vi "Drivebase Controller.vi"(8 "error in":errorcluster) -> ()   [LabVIEW 2019]
doc: "This VI executes continuously carrying out the current operation and responding to updates or new operations. It will often contain the timing or control code that is difficult to place directly in TeleOp. This VI generally opens all sensors and motors and isolates the rest of the robot code from knowing how the operations are carried out."
uses:
  <vilib>/Rock Robotics/WPI/Framework/Completion Status.ctl
  Drivebase Setpoints.ctl
  Drivebase Operations.ctl
  Bordeaux/bordeaux-pathinator/Bordeaux/Command Stuff/Single Cmd Info.ctl
  <vilib>/picture/picture.llb/imagedata.ctl
  <vilib>/Rock Robotics/WPI/ThirdParty/REV Robotics/SPARK MAX/Typedef/Spark MAX Idle Mode.ctl
  IMU/Typedef/ADIS16470 Data.ctl
  <vilib>/Rock Robotics/WPI/ThirdParty/REV Robotics/SPARK MAX/Typedef/Spark MAX Control Type.ctl
  Framework/Robot Global Data.vi
panel:
  out "x-y":u32(graph)
  out "timing delay err 2":dbl(graph)
  in  "Interactive Values":T1
  out "Current\nCmd":string
  in  "Buttons":cluster{"Execute Cmd":bool, "Abort Cmd":bool}
  out "Command Timing":cluster{"Start Time (ms)":u32, "Iterations":i32}
  out "Status":T5
  # "Tip: It may be helpful to observe inputs and sensor values.\nYou may also want to display tuning or debugging controls."
  # "Interactive Command: You may fill in the settings for a command\nand schedule it with the Execute button. You can observe and abort\nany command while fine tuning the code for the controller."
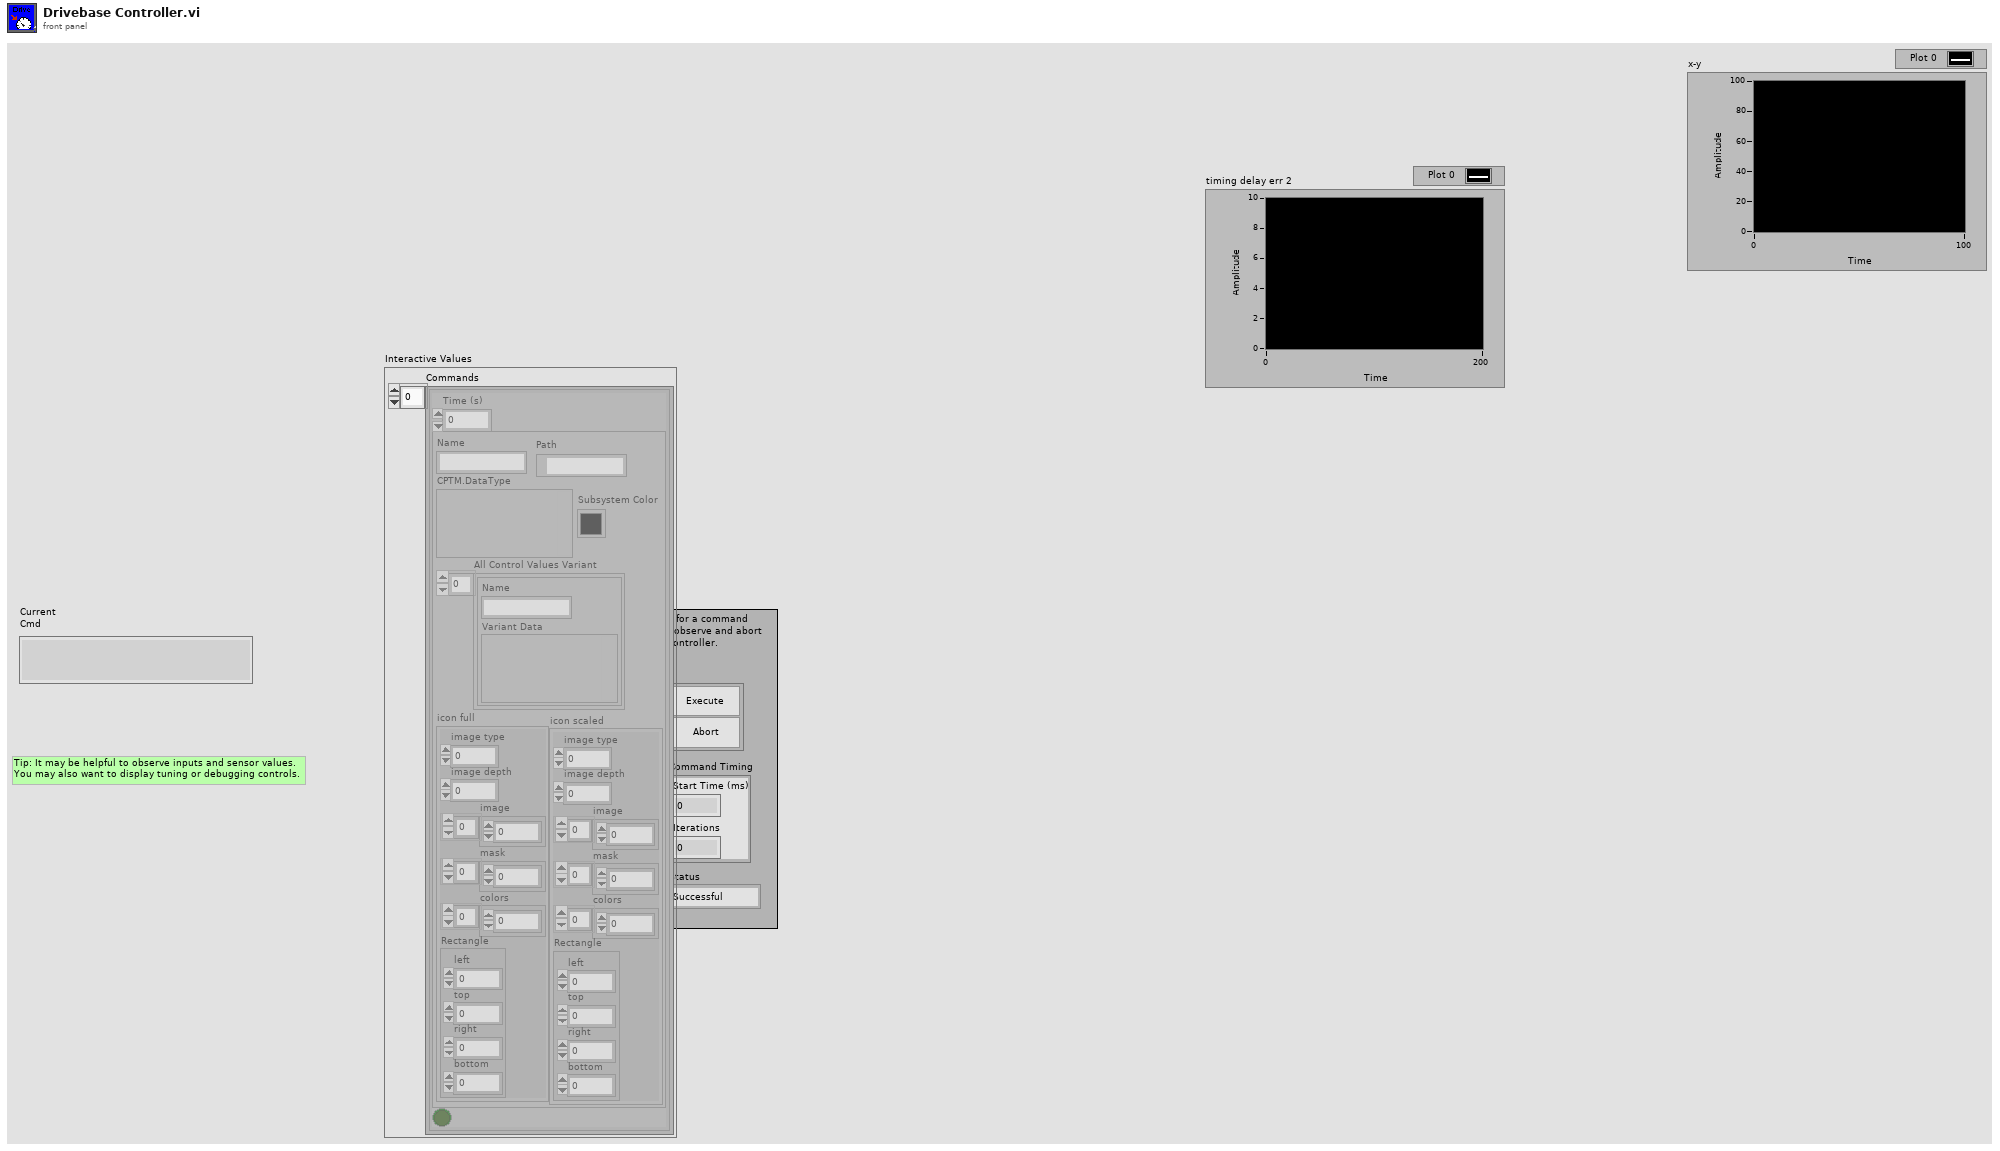
[diagram p1: front panel]
types:
  T1 = typedef "Drivebase Setpoints.ctl" = cluster{"Operation":T2, "Left Setpoint":dbl, "Right Setpoint":dbl, "Velocity":dbl[], "Angles":dbl[], "Reset Gyro":bool, "Booleans":cluster{"Robot Backwards":bool, "Path Backwards":bool}, "Commands":cluster{"Time (s)":dbl, T3, bool}[]}
  T2 = typedef "Drivebase Operations.ctl" = enum16{"Reserve", "Read Current", "Immediate", "Pathinator"}
  T3 = typedef "Single Cmd Info.ctl" = cluster{"Name":string, "CPTM.DataType":variant, "All Control Values Variant":cluster{"Name":string, "Variant Data":variant}[], "icon full":T4, "icon scaled":T4, "Path":path, "Subsystem Color":u32}
  T4 = typedef "imagedata.ctl" = cluster{"image type":i32, "image depth":i32, "image":u8[], "mask":u8[], "colors":u32[], "Rectangle":cluster{"left":i16, "top":i16, "right":i16, "bottom":i16}}
  T5 = typedef "Completion Status.ctl" = enum16{"Successful", "Aborted", "Incomplete"}
  T6 = cluster{"P Gain":dbl, "I Gain":dbl, "D Gain":dbl, "F Gain":dbl, "I Zone":dbl, "Min Output":dbl, "Max Output":dbl}
  T7 = typedef "Spark MAX Idle Mode.ctl" = enum16{"Coast", "Brake"}
  T8 = typedef "WPI_MotorControlDeviceRef.ctl" = cluster{"DeviceStatus":errorcluster, "Type":T9, "PWM":cluster{"PWM Channel":T10, "DeadBand":T11}, "CAN":cluster{"Device Number":u8, "SetOutput VI Ref":variant, "GetOutput VI Ref":variant, "Enable VI Ref":variant, "Disable VI Ref":variant, "Data":variant}, "Invert":bool, "DIO PWM":cluster{"PWM \"Enable\" Channel":T10, "DIOChannel":T12, "PWM Rate":dbl}}
  T9 = typedef "WPI_MotorControlType.ctl" = enum16{"PWM", "CAN", "DIO PWM"}
  T10 = typedef "FPGA_DIOPWMChannel.ctl" = enum8{"PWM 0", "PWM 1", "PWM 2", "PWM 3", "PWM 4", "PWM 5", "PWM 6", "PWM 7", "PWM 8", "PWM 9", "PWM MXP 0", "PWM MXP 1", "PWM MXP 2", "PWM MXP 3", "PWM MXP 4", "PWM MXP 5", "PWM MXP 6", "PWM MXP 7", "PWM MXP 8", "PWM MXP 9", "Invalid"}
  T11 = typedef "WPI_PWMDeadband.ctl" = cluster{"Name":string, "maxPositivePwm":i32, "minPositivePwm":i32, "centerPwm":i32, "maxNegativePwm":i32, "minNegativePwm":i32, "angularRange":u16}
  T12 = typedef "FPGA_DIOChannel.ctl" = enum8{"DIO 0", "DIO 1", "DIO 2", "DIO 3", "DIO 4", "DIO 5", "DIO 6", "DIO 7", "DIO 8", "DIO 9", "DIO MXP 0", "DIO MXP 1", "DIO MXP 2", "DIO MXP 3", "DIO MXP 4", "DIO MXP 5", "DIO MXP 6", "DIO MXP 7", "DIO MXP 8", "DIO MXP 9", "DIO MXP 10", "DIO MXP 11", "DIO MXP 12", "DIO MXP 13", "DIO MXP 14", "DIO MXP 15", "SPI Port CS1", "SPI Port CS2", "SPI Port CS3", "SPI Port MISO", "SPI Port MOSI", "Invalid"}
  T13 = typedef "ADIS16470 Device Reference.ctl" = cluster{"DevStatus":errorcluster, "Hardware Config":T14, "Calibration Complete":refnum<notifier>, "Status FIFO":refnum<k33>, "Last Value Reference":refnum<data-value>, "Sychronous Process VI":T17, "Cmd FIFO":refnum<k33>, "Source":T18, "Data FIFO":refnum<k33>, "Calibration Time":T22}
  T14 = typedef "ADIS16470 Hardware Configuration.ctl" = cluster{"SPI Clock Rate (Hz)":dbl, "IMU SPI Mode (3)":T15, "IMU Reset Pin":T12, "IMU SPI Bus":T16, "IMU Data Ready Pin":T12, "Stall Config":cluster{"Pow2BytesPerRead":u8, "StallTicks":u16, "CsToSclkTicks":u8}}
  T15 = typedef "WPI_SPIMode.ctl" = enum16{"Mode 0 (Clk Idle Low,Sample on Leading)", "Mode 1 (Clk Idle Low,Sample on Trailing)", "Mode 2 (Clk Idle High,Sample on Leading)", "Mode 3 (Clk Idle High,Sample on Trailing)"}
  T16 = typedef "spi_bus.ctl" = enum16{"SPI On-Board, CS0", "SPI On-Board, CS1", "SPI On-Board, CS2", "SPI On-Board, CS3", "SPI MXP", "Invalid"}
  T17 = typedef "ADIS16470 Process.ctl" = refnum<vi>
  T18 = typedef "FPGA_CounterEncoderSourceConvertionLVSourceType.ctl" = cluster{"DevStatus":errorcluster, "AnalogTriggerMode?":bool, "DigitalMode":cluster{"DIO Channel":T19}, "AnalogTriggerMode":cluster{"AnalogTriggerIndex":T20, "OutputType":T21}}
  T19 = typedef "FPGA_DIODigitalSourceChannel.ctl" = enum8{"DIO 0", "DIO 1", "DIO 2", "DIO 3", "DIO 4", "DIO 5", "DIO 6", "DIO 7", "DIO 8", "DIO 9", "DIO MXP 0", "DIO MXP 1", "DIO MXP 2", "DIO MXP 3", "DIO MXP 4", "DIO MXP 5", "DIO MXP 6", "DIO MXP 7", "DIO MXP 8", "DIO MXP 9", "DIO MXP 10", "DIO MXP 11", "DIO MXP 12", "DIO MXP 13", "DIO MXP 14", "DIO MXP 15", "SPI Port CS1", "SPI Port CS2", "SPI Port CS3", "SPI Port MISO", "SPI Port MOSI", "Disabled"}
  T20 = typedef "FPGA_AnalogTriggerIndex.ctl" = enum8{"Trig 0", "Trig 1", "Trig 2", "Trig 3", "Trig 4", "Trig 5", "Trig 6", "Trig 7", "Invalid"}
  T21 = typedef "FPGA_AnalogTriggerOutType.ctl" = enum16{"InWindow", "TriggerState", "Rising", "Falling"}
  T22 = typedef "ADIS16470 Calibration Time.ctl" = enum16{"32ms", "64ms", "128ms", "256ms", "512ms", "1s", "2s", "4s", "8s", "16s", "32s", "64s"}
  T23 = typedef "Command Status Info.ctl" = cluster{"Name":string, "Status":T5, "notifier out":T24}
  T24 = typedef "Completion Notifier.ctl" = refnum<notifier>
  T25 = cluster{"Current Command":T1, "Command Timing":cluster{"Start Time (ms)":u32, "Iterations":i32}, "Command Arguments":cluster{"Command Info":T23, "Description":string, "Default Command":T1, "queue out":refnum<queue>, "Subsystem Name":string}}
  T26 = typedef "ADIS16470 Data.ctl" = cluster{"XAngle":dbl, "YAngle":dbl, "ZAngle":dbl}
  T27 = typedef "Spark MAX Control Type.ctl" = enum16{"Percent VBus", "Voltage", "Velocity", "Position", "Smart Motion", "Current", "Smart Velocity"}
  T28 = cluster{"Robot Backwards":bool, "Path Backwards":bool}
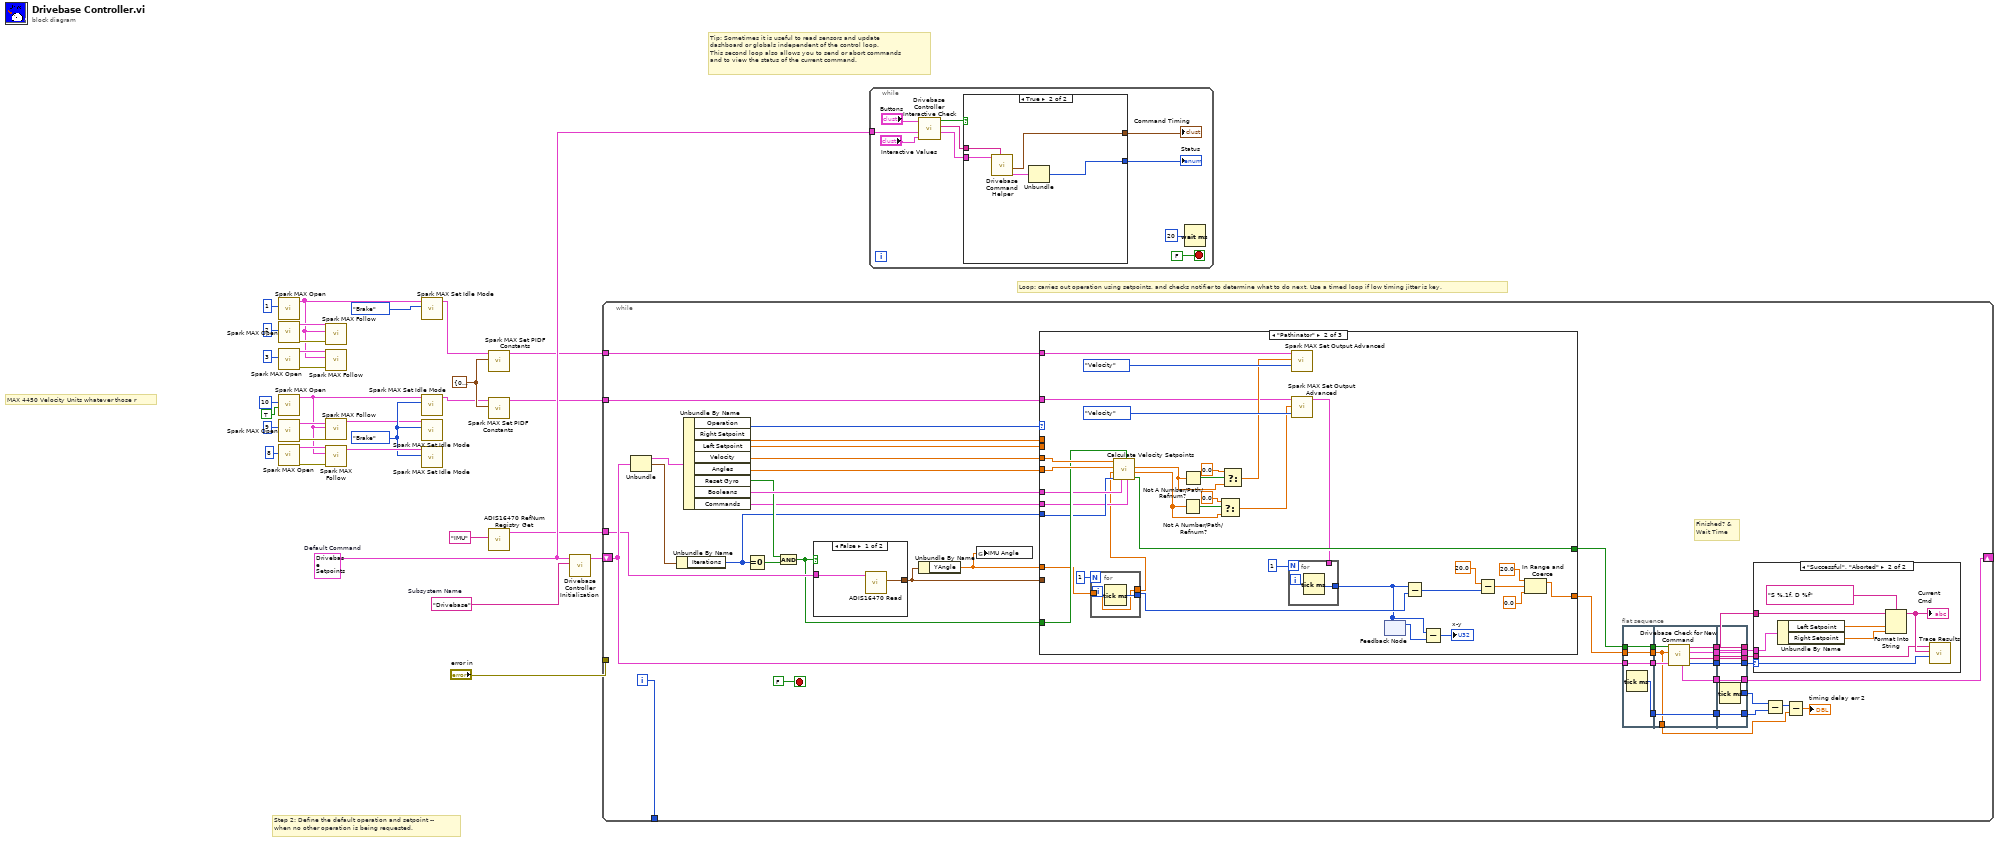
[diagram p0: block diagram]
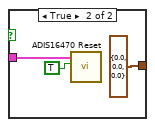
[diagram p2: hidden frame]
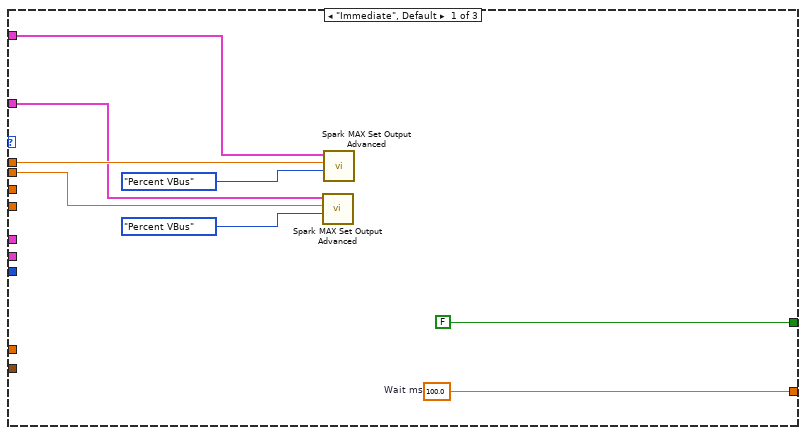
[diagram p3: hidden frame]
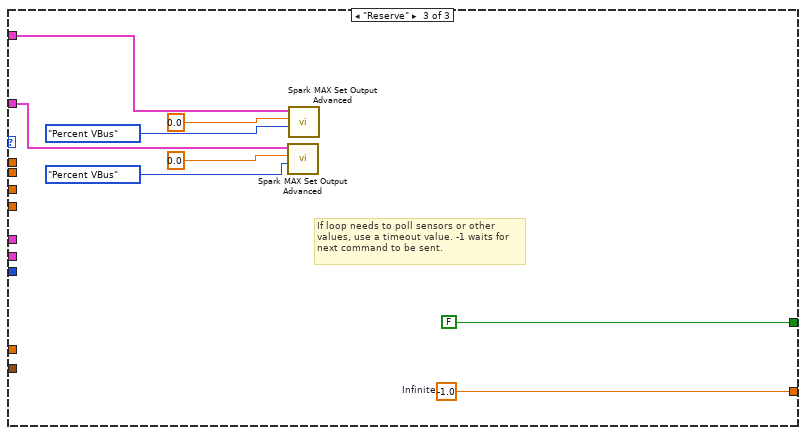
[diagram p4: hidden frame]
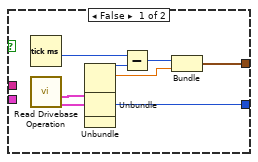
[diagram p6: hidden frame]
diagram:
  w7 = T6 {"P Gain"=0.0003, "I Gain"=1e-09, "D Gain"=0.0, "F Gain"=0.0002, "I Zone"=0.0, "Min Output"=-1.0, "Max Output"=1.0} ("PID Constants")
  w8 = Spark_MAX_Idle_Mode."Brake" ("Idle Mode")
  w29 = T1 {"Operation"=enum."Reserve", "Left Setpoint"=0.0, "Right Setpoint"=0.0, "Velocity"=[], "Angles"=[], "Reset Gyro"=FALSE, "Booleans"={"Robot Backwards"=FALSE, "Path Backwards"=FALSE}, "Commands"=[]}  # Default Command
  w30 = "Drivebase"  # Subsystem Name
  # "MAX 4450 Velocity Units whatever those r"
  # "Tip: Sometimes it is useful to read sensors and update\ndashboard or globals independent of the control loop.\nThis second loop also allows you to send or abort commands\nand to view the status of the current command."
  # "Step 2: Define the default operation and setpoint --\nwhen no other operation is being requested."
  # "Loop: carries out operation using setpoints, and checks notifier to determine what to do next. Use a timed loop if low timing jitter is key."
  n1 = call <vilib>:"Spark MAX Open.vi"("Device Number"=u8 1) -> ("MotorControlDeviceRef"=w11:T8)  [unwired: 9 in, 1 out]
  n2 = call <vilib>:"Spark MAX Open.vi"("Device Number"=u8 2) -> ("error out"=w20:errorcluster, "MotorControlDeviceRef"=w21:T8)  [unwired: 9 in]
  n3 = call <vilib>:"Spark MAX Open.vi"("Device Number"=u8 3) -> ("error out"=w22:errorcluster, "MotorControlDeviceRef"=w23:T8)  [unwired: 9 in]
  n4 = call <vilib>:"Spark MAX Open.vi"("Invert"=TRUE, "Device Number"=u8 10) -> ("MotorControlDeviceRef"=w2:T8)  [unwired: 8 in, 1 out]
  n5 = call <vilib>:"Spark MAX Open.vi"("Device Number"=u8 9) -> ("error out"=w18:errorcluster, "MotorControlDeviceRef"=w17:T8)  [unwired: 9 in]
  n6 = call <vilib>:"Spark MAX Open.vi"("Device Number"=u8 8) -> ("error out"=w16:errorcluster, "MotorControlDeviceRef"=w15:T8)  [unwired: 9 in]
  n7 = call <vilib>:"Spark MAX Follow.vi"("error in (no error)"=w20, "Master Controller"=w11, "MotorControlDeviceRef"=w21) -> ()  [unwired: 7 in, 2 out]
  n8 = call <vilib>:"Spark MAX Follow.vi"("error in (no error)"=w22, "Master Controller"=w11, "MotorControlDeviceRef"=w23) -> ()  [unwired: 7 in, 2 out]
  n9 = call <vilib>:"Spark MAX Follow.vi"("error in (no error)"=w18, "Master Controller"=w2, "MotorControlDeviceRef"=w17) -> ("MotorControlDeviceRef"=w3:T8)  [unwired: 7 in, 1 out]
  n10 = call <vilib>:"Spark MAX Follow.vi"("error in (no error)"=w16, "Master Controller"=w2, "MotorControlDeviceRef"=w15) -> ("MotorControlDeviceRef"=w9:T8)  [unwired: 7 in, 1 out]
  n11 = call <vilib>:"Spark MAX Set Idle Mode.vi"("Idle Mode"=Spark_MAX_Idle_Mode."Brake", "MotorControlDeviceRef in"=w11) -> ("MotorControlDeviceRef out"=w6:T8)  [unwired: 8 in, 1 out]
  n12 = call <vilib>:"Spark MAX Set Idle Mode.vi"("Idle Mode"=w8, "MotorControlDeviceRef in"=w2) -> ("MotorControlDeviceRef out"=w1:T8)  [unwired: 8 in, 1 out]
  n13 = call <vilib>:"Spark MAX Set Idle Mode.vi"("Idle Mode"=w8, "MotorControlDeviceRef in"=w3) -> ()  [unwired: 8 in, 2 out]
  n14 = call <vilib>:"Spark MAX Set Idle Mode.vi"("Idle Mode"=w8, "MotorControlDeviceRef in"=w9) -> ()  [unwired: 8 in, 2 out]
  n15 = call <vilib>:"Spark MAX Set PIDF Constants.vi"("PID Constants"=w7, "MotorControlDeviceRef"=w6) -> ("MotorControlDeviceRef"=w4:T8)  [unwired: 8 in, 1 out]
  n16 = call <vilib>:"Spark MAX Set PIDF Constants.vi"("PID Constants"=w7, "MotorControlDeviceRef"=w1) -> ("MotorControlDeviceRef"=w5:T8)  [unwired: 8 in, 1 out]
  n17 = call "ADIS16470 RefNum Registry Get.vi"("refnum name"="IMU") -> ("ADIS16470DevRef out"=w28:T13)  [unwired: 9 in, 1 out]
  n18 = call "Drivebase Controller Initialization.vi"("Subsystem Name"=w30, "Default Command"=w29) -> ("Current Command"=w31:T25)  [unwired: 9 in]
  n19 = while {
    shift-right: [w68] -> _
    shift-left: w31 -> [w61]
    tunnel: [w74] -> _
    tunnel: "error in" -> [_]
    tunnel: w28 -> [w53]
    tunnel: w5 -> [w57]
    tunnel: w4 -> [w56]
    i -> [w74]
    stop <- FALSE stop-if-true
    # "Finished? &\nWait Time"
    n20 = Unbundle(w61) -> ("Current Command"=w73:T1, "Command Timing"=w70:cluster{"Start Time (ms)":u32, "Iterations":i32})  [unwired: 1 out]
    n21 = Unbundle By Name(w70) -> ("Iterations"=w51:i32)
    n22 = Unbundle By Name(w73) -> ("Operation"=w72:T2, "Right Setpoint"=w71:dbl, "Left Setpoint"=w69:dbl, "Velocity"=w60:dbl[], "Angles"=w59:dbl[], "Reset Gyro"=w54:bool, "Booleans"=w58:T28, "Commands"=w48:cluster{"Time (s)":dbl, T3, bool}[])
    n23 = Equal To 0?(x=w51) -> (x = 0?=w55:bool)
    n24 = And(x=w54, y=w55) -> (x .and. y?=w52:bool)
    n25 = case shown="False" w52 {
      tunnel: w53 -> [w97 w100]
      tunnel: [w96 T26 {"XAngle"=0.0, "YAngle"=0.0, "ZAngle"=0.0} ("ADIS16470 Value")] -> w50
      frame False {
        n26 = call "ADIS16470 Read.vi"("ADIS16470DevRef"=w97) -> ("ADIS16470 Value"=w96:T26)  [unwired: 7 in, 3 out]
      }
      frame True {
        n27 = call "ADIS16470 Reset.vi"("Reset?"=TRUE, "ADIS16470DevRef"=w100) -> ()  [unwired: 8 in, 2 out]
      }
    }
    n28 = Unbundle By Name(w50) -> ("YAngle"=w49:dbl)
    n29 = global write "Robot Global Data.vi" "IMU Angle"(w49) -> ()
    n30 = case shown="\"Pathinator\"" w72 {
      tunnel: [w108 w109 w153] -> w66
      tunnel: [FALSE ("ignore previous (F)") w132 FALSE ("ignore previous (F)")] -> w67
      tunnel: w71 -> [w103 _ _]
      tunnel: w69 -> [w107 _ _]
      tunnel: w60 -> [_ w140 _]
      tunnel: w59 -> [_ w139 _]
      tunnel: w58 -> [_ w126 _]
      tunnel: w57 -> [w102 w128 w146]
      tunnel: w56 -> [w101 w129 w147]
      tunnel: w49 -> [_ w120 _]
      tunnel: w52 -> [_ w127 _]
      tunnel: w51 -> [_ w125 _]
      tunnel: w50 -> [_ _ _]
      tunnel: w48 -> [_ w123 _]
      frame "Immediate", Default {
        w108 = 100.0  # Wait ms
        n31 = call <vilib>:"Spark MAX Set Output Advanced.vi"("Control Mode"=Spark_MAX_Control_Type."Percent VBus", "Setpoint"=w107, "MotorControlDevRef"=w102) -> ()  [unwired: 7 in, 2 out]
        n32 = call <vilib>:"Spark MAX Set Output Advanced.vi"("Control Mode"=Spark_MAX_Control_Type."Percent VBus", "Setpoint"=w103, "MotorControlDevRef"=w101) -> ()  [unwired: 7 in, 2 out]
      }
      frame "Pathinator" {
        n33 = for {
          N: 1 -> [_]
          tunnel: [w144] -> w118
          tunnel: w120 -> [w143]
          tunnel: [w143] -> w119
          n34 = Tick Count (ms)() -> (millisecond timer value=w144:u32)
        }
        n35 = call "Calculate Velocity Setpoints.vi"("Commands"=w123, "Reset Accumulator"=w127, "Booleans"=w126, "Iterations"=w125, "IMU"=w119, "Angles"=w139, "Velocity"=w140) -> ("Finished"=w132:bool, "Left Velocity"=w124:dbl, "Right Velocity"=w134:dbl)  [unwired: 2 in]
        n36 = Not A Number/Path/Refnum?(number/path/refnum=w124) -> (NaN/Path/Refnum?=w137:bool)
        n37 = Not A Number/Path/Refnum?(number/path/refnum=w134) -> (NaN/Path/Refnum?=w138:bool)
        n38 = Select(t=0.0, s=w137, f=w124) -> (s? t:f=w130:dbl)
        n39 = Select(t=0.0, s=w138, f=w134) -> (s? t:f=w131:dbl)
        n40 = call <vilib>:"Spark MAX Set Output Advanced.vi"("Control Mode"=Spark_MAX_Control_Type."Velocity", "Setpoint"=w131, "MotorControlDevRef"=w129) -> ()  [unwired: 7 in, 2 out]
        n41 = call <vilib>:"Spark MAX Set Output Advanced.vi"("Control Mode"=Spark_MAX_Control_Type."Velocity", "Setpoint"=w130, "MotorControlDevRef"=w128) -> ("MotorControlDevRef"=w122:T8)  [unwired: 7 in, 1 out]
        n42 = for {
          N: 1 -> [_]
          tunnel: [w145] -> w114
          tunnel: w122 -> [_]
          n43 = Tick Count (ms)() -> (millisecond timer value=w145:u32)
        }
        n44 = feedback-in #1(w114) -> ()
        n45 = feedback #1() -> (w115:u32)  [unwired: 1 in]
        n46 = Subtract(x=w114, y=w118) -> (x-y=w116:u32)
        n47 = Subtract(x=w114, y=w115) -> (x-y=→"x-y":u32)
        n48 = Subtract(x=20.0, y=w116) -> (x-y=w110:dbl)
        n49 = In Range and Coerce(upper limit=20.0, x=w110, lower limit=0.0) -> (coerced(x)=w109:dbl)  [unwired: 1 out]
      }
      frame "Reserve" {
        w153 = -1.0  # Infinite
        # "If loop needs to poll sensors or other\nvalues, use a timeout value. -1 waits for\nnext command to be sent."
        n50 = call <vilib>:"Spark MAX Set Output Advanced.vi"("Control Mode"=Spark_MAX_Control_Type."Percent VBus", "Setpoint"=0.0, "MotorControlDevRef"=w146) -> ()  [unwired: 7 in, 2 out]
        n51 = call <vilib>:"Spark MAX Set Output Advanced.vi"("Control Mode"=Spark_MAX_Control_Type."Percent VBus", "Setpoint"=0.0, "MotorControlDevRef"=w147) -> ()  [unwired: 7 in, 2 out]
      }
    }
    n52 = flat-sequence {
      tunnel: w61 -> [w77]
      tunnel: w66 -> [w78]
      tunnel: w67 -> [w79]
      tunnel: [w79] -> w42
      tunnel: [w78] -> w41
      tunnel: [w77] -> w40
      tunnel: [w76] -> w38
      tunnel: [w88] -> w47
      tunnel: [w86] -> w46
      tunnel: [w85] -> w45
      tunnel: [w84] -> w44
      tunnel: [w83] -> w43
      tunnel: w42 -> [w87]
      tunnel: w41 -> [w80]
      tunnel: w40 -> [w82]
      tunnel: w38 -> [w81]
      tunnel: [w81] -> w37
      tunnel: [w80] -> w34
      tunnel: [w91] -> w62
      tunnel: [w92] -> w63
      tunnel: [w93] -> w64
      tunnel: [w94] -> w65
      tunnel: [w95] -> w68
      tunnel: w47 -> [w95]
      tunnel: w46 -> [w94]
      tunnel: w45 -> [w93]
      tunnel: w44 -> [w92]
      tunnel: w43 -> [w91]
      tunnel: [w90] -> w39
      tunnel: w37 -> [w89]
      tunnel: [w89] -> w36
      frame #0 {
        n53 = Tick Count (ms)() -> (millisecond timer value=w76:u32)
      }
      frame #1 {
        n54 = call "Drivebase Check for New Command.vi"("Current Command"=w82, "Wait time (ms)"=w80, "Finished?"=w87) -> ("Completion"=w83:T5, "Subsystem Name"=w84:string, "Current Command"=w85:T1, "Initial Trace String"=w86:string, "NextCommand"=w88:T25)  [unwired: 4 in]
      }
      frame #2 {
        n55 = Tick Count (ms)() -> (millisecond timer value=w90:u32)
      }
    }
    n56 = case shown="\"Successful\", \"Aborted\"" w62 {
      selector: w62 -> [_ w161]
      tunnel: w65 -> [_ w157]
      tunnel: w64 -> [_ w158]
      tunnel: w63 -> [_ w154]
      frame "Incomplete", Default {
        # "Continuing current command"
      }
      frame "Successful", "Aborted" {
        # "Report and setup for next command"
        n57 = Unbundle By Name(w158) -> ("Left Setpoint"=w160:dbl, "Right Setpoint"=w155:dbl)
        n58 = Format Into String(format string="S %.1f, D %f", initial string=w157, w160, w155) -> (resulting string=w156:string)  [unwired: 1 in, 1 out]
        "Current\nCmd" <- w156
        n59 = call <vilib>:"Trace Results.vi"("Status of previous command"=w161, "Description"=w156, "Subsystem"=w154) -> ()  [unwired: 9 in]
      }
    }
    n60 = Subtract(x=w39, y=w36) -> (x-y=w35:u32)
    n61 = Subtract(x=w35, y=w34) -> (x-y=→"timing delay err 2":dbl)
  }
  n62 = while {
    tunnel: w29 -> [w168]
    stop <- FALSE stop-if-true
    n63 = call "Drivebase Controller Interactive Check.vi"("Interactive Command in"="Interactive Values", "Default Command"=w168, "Buttons"="Buttons") -> ("Interactive Command out"=w165:T1, "Trace String"=w166:string, "Schedule"=w167:bool)  [unwired: 6 in]
    n64 = case shown="True" w167 {
      tunnel: [w179 w184] -> w164
      tunnel: w165 -> [_ w182]
      tunnel: [w175 w180] -> w163
      tunnel: w166 -> [_ w183]
      frame False {
        n65 = Tick Count (ms)() -> (millisecond timer value=w174:u32)
        n66 = call "Read Drivebase Operation.vi"() -> ("Command Info"=w172:T23, "SubSystem Data"=w173:T1)  [unwired: 9 in, 1 out]
        n67 = Unbundle(w173) -> ("Operation"=w178:T2, "Left Setpoint"=w176:dbl)  [unwired: 6 out]
        n68 = Unbundle(w172) -> ("Status"=w179:T5)  [unwired: 2 out]
        n69 = Subtract(x=w174, y=w178) -> (x-y=w177:u32)
        n70 = Bundle(w177, "Left Setpoint"=w176) -> (w175:cluster{u32, "Left Setpoint":dbl})  [unwired: 1 in]
      }
      frame True {
        n71 = call "Drivebase Command Helper.vi"("Description"=w183, "SubSystem Data"=w182) -> ("Command Info Out"=w181:T23, "Command Timing"=w180:cluster{"Start Time (ms)":u32, "Iterations":i32})  [unwired: 7 in, 1 out]
        n72 = Unbundle(w181) -> ("Status"=w184:T5)  [unwired: 2 out]
      }
    }
    "Status" <- w164
    "Command Timing" <- w163
    n73 = Wait (ms)(milliseconds to wait=u32 20) -> ()  [unwired: 1 out]
  }
